vi "MLSD Data to Dir-File Info.vi"(8 "error in (no error)":errorcluster, 10 "Data":string, 11 "FTP in":refnum<class "FTP.lvclass">) -> (0 "error out":errorcluster, 2 "Dir-File Info":T1, 3 "FTP out":refnum<class "FTP.lvclass">)   [LabVIEW 2014, in "FTP.lvlib" / "FTP.lvclass"]
uses:
  FTP.lvclass
  controls/Dir-File Info.ctl
  controls/Dir-File Type.ctl
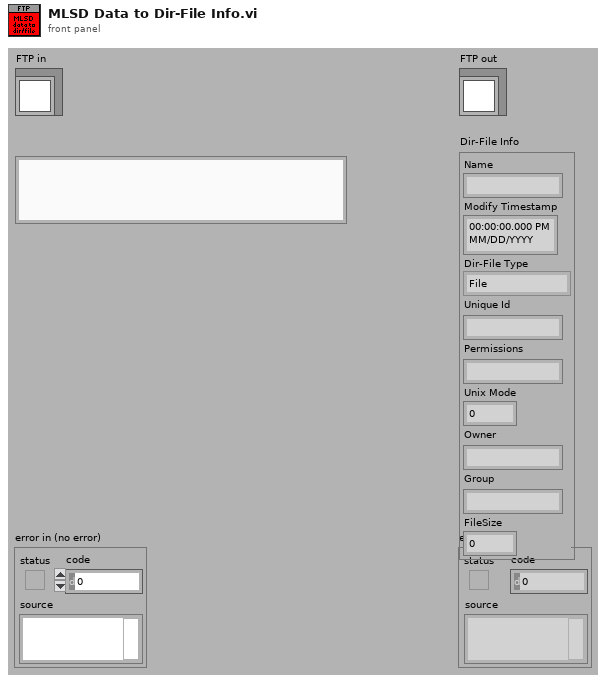
[diagram p1: front panel]
types:
  T1 = typedef "FTP.lvlib/FTP.lvclass/Dir-File Info.ctl" = cluster{"Name":string, "Modify Timestamp":timestamp, "Dir-File Type":T2, "Unique Id":string, "Permissions":string, "Unix Mode":u16, "Owner":string, "Group":string, "FileSize":i64}
  T2 = typedef "FTP.lvlib/FTP.lvclass/Dir-File Type.ctl" = enum16{"File", "Listed Directory", "Parent Directory", "Directory", "Unknown"}
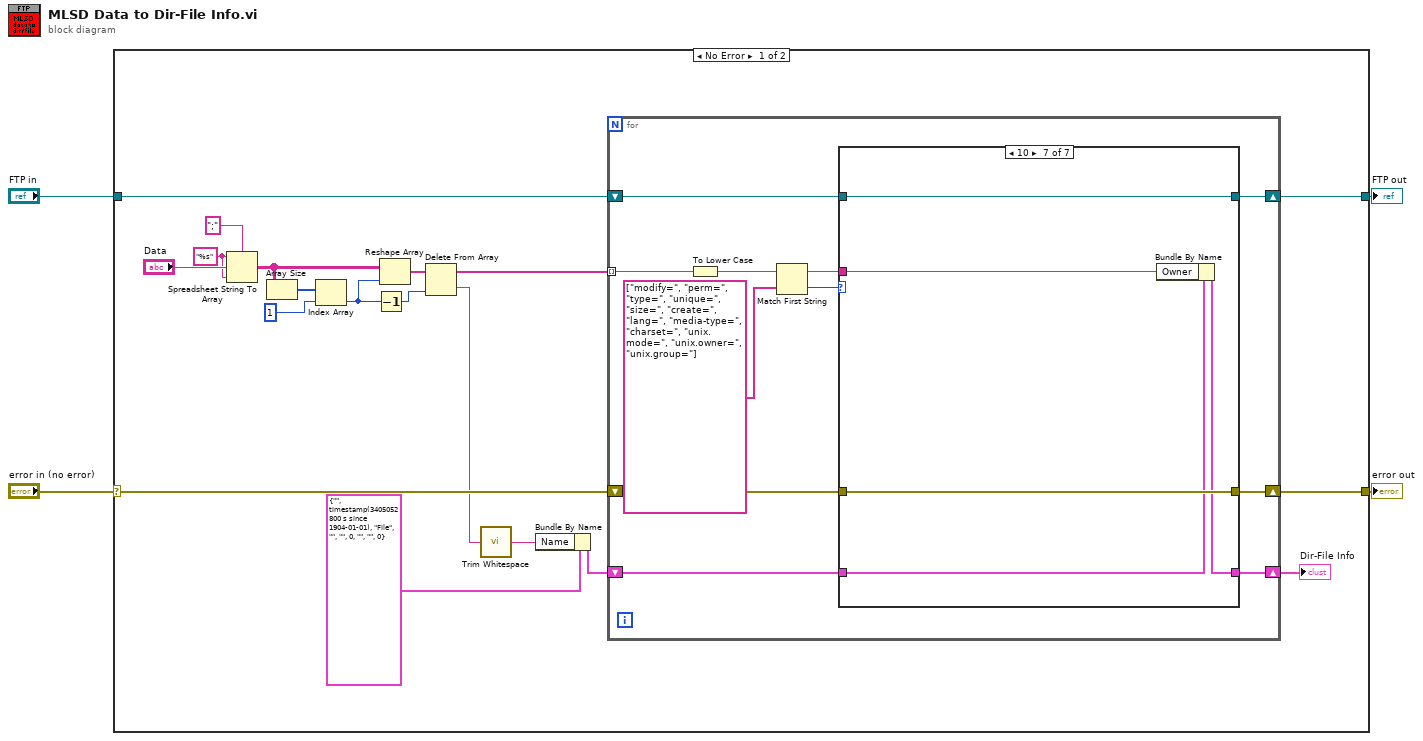
[diagram p0: block diagram]
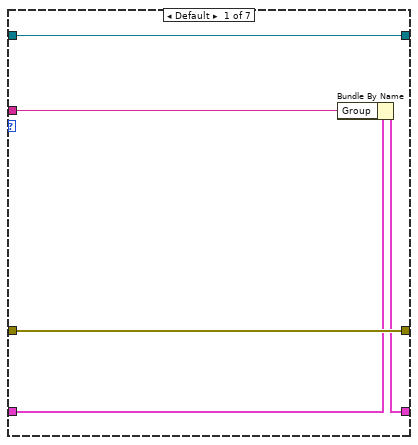
[diagram p2: hidden frame]
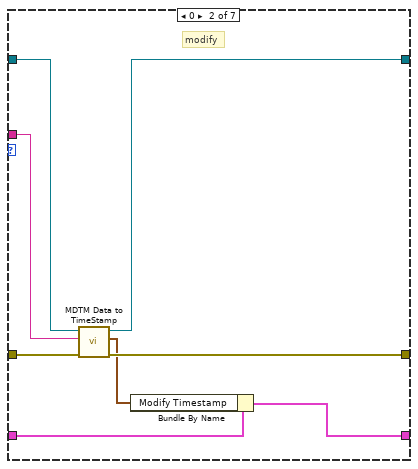
[diagram p3: hidden frame]
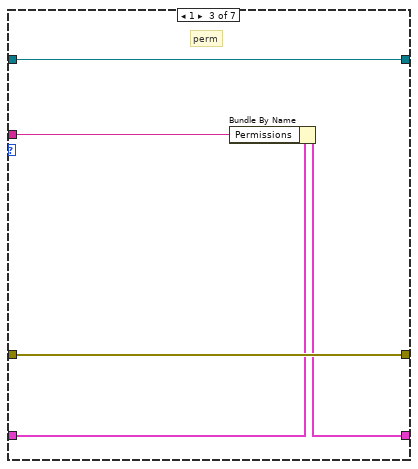
[diagram p4: hidden frame]
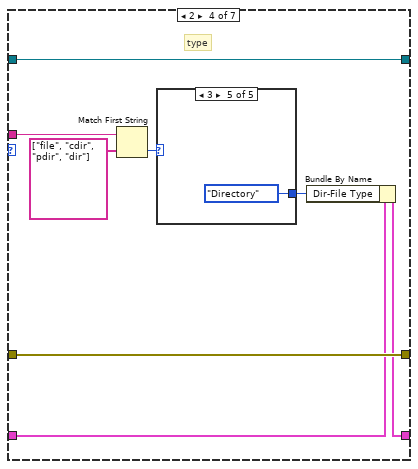
[diagram p5: hidden frame]
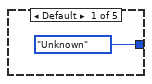
[diagram p6: hidden frame]
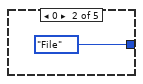
[diagram p7: hidden frame]
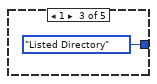
[diagram p8: hidden frame]
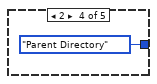
[diagram p9: hidden frame]
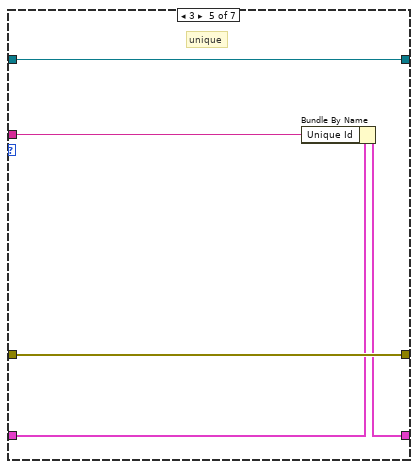
[diagram p10: hidden frame]
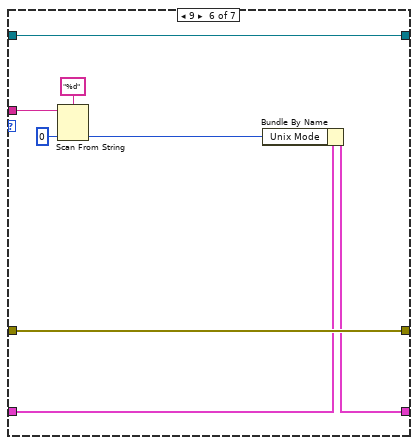
[diagram p11: hidden frame]
diagram:
  n1 = case shown="No Error" "error in (no error)" {
    selector: "error in (no error)" -> [w20 w85]
    tunnel: [w19 w85] -> w3
    tunnel: [w9 w84] -> w1
    tunnel: "FTP in" -> [w10 w84]
    frame No Error {
      w21 = "%s" ("format string")
      n2 = Spreadsheet String To Array(delimiter (Tab)=";", format string=w21, spreadsheet string="Data", array type (2D Dbl)=w21) -> (array=w18:string[][])
      n3 = Array Size(array=w18) -> (size(s)=w17:i32[])
      n4 = Index Array(array=w17, index=1) -> (element=w12:i32)
      n5 = Decrement(x=w12) -> (x-1=w13:i32)
      n6 = Reshape Array(w18, w12) -> (w15:string[])
      n7 = Delete From Array(array=w15, index=w13) -> (deleted portion=w11:string, array with subset deleted=w14:string[])  [unwired: 1 in]
      n8 = call <vilib>:"Trim Whitespace.vi"("string"=w11) -> ("trimmed string"=w5:string)  [unwired: 1 in]
      n9 = Bundle By Name(cluster=T1 {"Name"="", "Modify Timestamp"=timestamp(3405052800 s since 1904-01-01), "Dir-File Type"=enum."File", "Unique Id"="", "Permissions"="", "Unix Mode"=0, "Owner"="", "Group"="", "FileSize"=0} ("Dir-File Info"), "Name"=w5) -> (w6:T1)
      n10 = for {
        shift-right: [w31] -> w19
        shift-left: w20 -> [w32]
        tunnel: w14 -> [w34] mode=indexing
        shift-right: [w27] -> w9
        shift-left: w10 -> [w28]
        shift-right: [w25] -> w7
        shift-left: w6 -> [w26]
        n11 = To Lower Case(string=w34) -> (all lower case string=w24:string)
        n12 = Match First String(2:string[] ["modify=", "perm=", "type=", "unique=", "size=", "create=", "lang=", "media-type=", "charset=", "unix.mode=", "unix.owner=", "unix.group="] ("operators (none)"), 3:w24) -> (0:w33:i32, 1:w30:string)
        n13 = case shown="10" w33 {
          tunnel: w32 -> [w39 w47 w52 w60 w70 w74 w83]
          tunnel: [w39 w46 w52 w60 w70 w74 w83] -> w31
          tunnel: w30 -> [w35 w43 w48 w56 w66 w77 w79]
          tunnel: w28 -> [w38 w45 w51 w59 w69 w78 w82]
          tunnel: [w38 w44 w51 w59 w69 w78 w82] -> w27
          tunnel: w26 -> [w37 w42 w50 w58 w68 w73 w81]
          tunnel: [w36 w40 w49 w57 w67 w72 w80] -> w25
          frame Default {
            n14 = Bundle By Name(cluster=w37, "Group"=w35) -> (w36:T1)
          }
          frame 0 {
            # "modify"
            n15 = call "MDTM Data to TimeStamp.vi"("error in (no error)"=w47, "MDTM Data"=w43, "FTP in"=w45) -> ("error out"=w46:errorcluster, "time stamp"=w41:timestamp, "FTP out"=w44:refnum<class "FTP.lvclass">)  [unwired: 6 in]
            n16 = Bundle By Name(cluster=w42, "Modify Timestamp"=w41) -> (w40:T1)
          }
          frame 1 {
            # "perm"
            n17 = Bundle By Name(cluster=w50, "Permissions"=w48) -> (w49:T1)
          }
          frame 2 {
            # "type"
            n18 = Match First String(2:string[] ["file", "cdir", "pdir", "dir"] ("string array"), 3:w56) -> (0:w54:i32)  [unwired: 1 out]
            n19 = case shown="3" w54 {
              tunnel: [Dir-File_Type."Unknown" ("Dir-File Type") Dir-File_Type."File" ("Dir-File Type") Dir-File_Type."Listed Directory" ("Dir-File Type") Dir-File_Type."Parent Directory" ("Dir-File Type") Dir-File_Type."Directory" ("Dir-File Type")] -> w53
              frame Default {
              }
              frame 0 {
              }
              frame 1 {
              }
              frame 2 {
              }
              frame 3 {
              }
            }
            n20 = Bundle By Name(cluster=w58, "Dir-File Type"=w53) -> (w57:T1)
          }
          frame 3 {
            # "unique"
            n21 = Bundle By Name(cluster=w68, "Unique Id"=w66) -> (w67:T1)
          }
          frame 9 {
            n22 = Scan From String(format string="%d", input string=w77, default 1=u16 0 ("default value 1")) -> (output 1=w71:u16)  [unwired: 2 in, 3 out]
            n23 = Bundle By Name(cluster=w73, "Unix Mode"=w71) -> (w72:T1)
          }
          frame 10 {
            n24 = Bundle By Name(cluster=w81, "Owner"=w79) -> (w80:T1)
          }
        }
      }
      "Dir-File Info" <- w7
    }
    frame Error {
    }
  }
  "error out" <- w3
  "FTP out" <- w1
